vi "Generate Observed Sequence.vi"(9 "Length of observation":i32, 11 "HMM Cluster":T1) -> (3 "Observed states":i32[](array[numeric]))   [LabVIEW 2014, in "HMM.lvlib"]
doc: "Generates a sequence of observed states based on the HMM lambda."
uses:
  HMM.lvlib
  Control/HMM Cluster.ctl
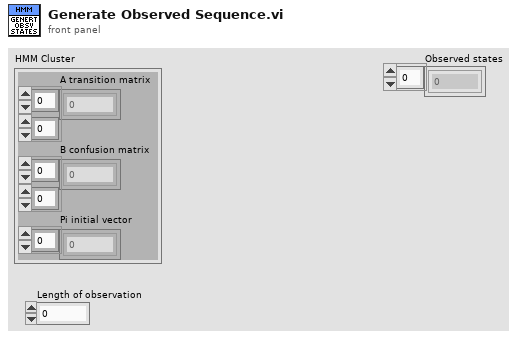
[diagram p1: front panel]
types:
  T1 = typedef "HMM.lvlib/HMM Cluster.ctl" = cluster{"A transition matrix":dbl[][], "B confusion matrix":dbl[][], "Pi initial vector":dbl[]}
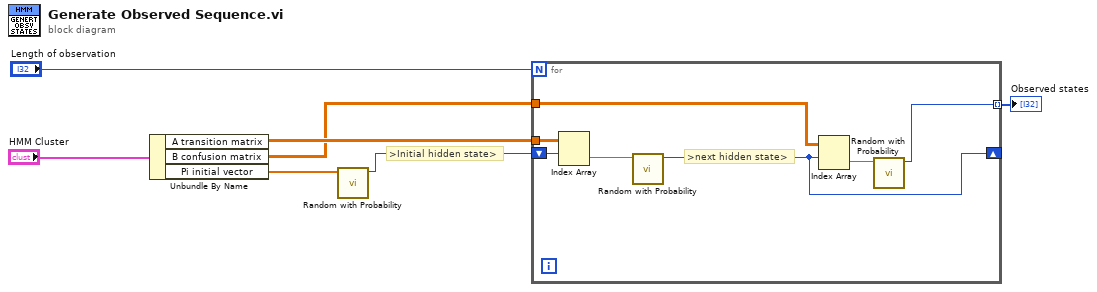
[diagram p0: block diagram]
diagram:
  # ">Initial hidden state>"
  n1 = Unbundle By Name("HMM Cluster") -> ("A transition matrix"=w6:dbl[][], "B confusion matrix"=w4:dbl[][], "Pi initial vector"=w7:dbl[])
  n2 = call "Random with Probability.vi"("Probability"=w7) -> ("Class"=w5:i32)  [unwired: 10 in]
  n3 = for {
    N: "Length of observation" -> [_]
    tunnel: w6 -> [w14]
    tunnel: w4 -> [w11]
    shift-right: [w9] -> _
    shift-left: w5 -> [w13]
    tunnel: [w8] -> w2 mode=indexing
    # ">next hidden state>"
    n4 = Index Array(array=w14, index (row)=w13) -> (element=w12:dbl[])  [unwired: 1 in]
    n5 = call "Random with Probability.vi"("Probability"=w12) -> ("Class"=w9:i32)  [unwired: 10 in]
    n6 = Index Array(array=w11, index (row)=w9) -> (element=w10:dbl[])  [unwired: 1 in]
    n7 = call "Random with Probability.vi"("Probability"=w10) -> ("Class"=w8:i32)  [unwired: 10 in]
  }
  "Observed states" <- w2
